vi "Read Setpoint.vi"(8 "error in":errorcluster, 11 "Alicat Controller in":refnum<class "Alicat Controller.lvclass">) -> (0 "error out":errorcluster, 1 "SPStr":string, 2 "Setpoint":sgl, 3 "Alicat Controller out":refnum<class "Alicat Controller.lvclass">)   [LabVIEW 2014, in "Alicat.lvlib" / "Alicat Controller.lvclass"]
doc: "Retrieve the setpoint from the private data cluster."
uses:
  Alicat Controller.lvclass
  Alicat Controller.lvclass/Alicat Controller.ctl
  Alicat.lvclass
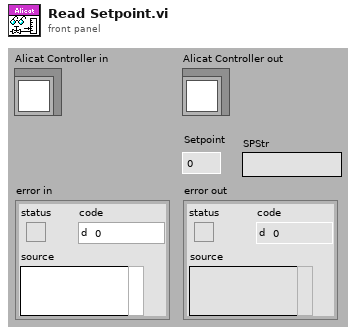
[diagram p1: front panel]
types:
  T1 = typedef "Alicat.lvlib/Alicat.lvclass/CtlSetup.ctl" = cluster{"Name":string, "Address":string, "fullScale":dbl, "Gas":T2}
  T2 = typedef "Alicat.lvlib/Alicat.lvclass/Gas.ctl" = enum16{"Air", "Ar", "CH4", "CO", "CO2", "C2H6", "H2", "He", "N2", "NO", "Ne", "O2", "C3H8", "n-C4H10", "C2H2", "C2H4", "i-C2H10", "Kr", "Xe"}
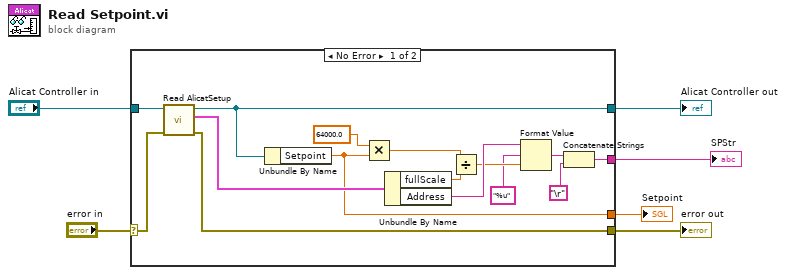
[diagram p0: block diagram]
diagram:
  n1 = case shown="No Error" "error in" {
    selector: "error in" -> [w8 w23]
    tunnel: [w7 w23] -> w5
    tunnel: [w11 w22] -> w3
    tunnel: "Alicat Controller in" -> [w13 w22]
    tunnel: [w10 _] -> w2
    tunnel: [w9 _] -> w1
    frame No Error {
      n2 = call "Read AlicatSetup.vi"("error in (no error)"=w8, "Alicat in"=w13) -> ("error out"=w7:errorcluster, "AlicatSetup"=w12:T1, "Alicat out"=w11:refnum<class "Alicat Controller.lvclass">)  [unwired: 7 in]
      n3 = Unbundle By Name(w11) -> ("Setpoint"=w9:sgl)
      n4 = Multiply(x=sgl 64000.0, y=w9) -> (x*y=w16:sgl)
      n5 = Unbundle By Name(w12) -> ("fullScale"=w15:dbl, "Address"=w21:string)
      n6 = Divide(x=w16, y=w15) -> (x/y=w20:dbl)
      n7 = Format Value(string ("")=w21, format string="%u", value (0)=w20) -> (output string=w18:string)
      n8 = Concatenate Strings(w18, "\r" ("string")) -> (w10:string)
    }
    frame Error {
    }
  }
  "error out" <- w5
  "Alicat Controller out" <- w3
  "Setpoint" <- w1
  "SPStr" <- w2
